vi "Date Start (000000).vi"(11 "Datetime":timestamp) -> (1 "檔名":string, 3 "Date + 00:00:00":timestamp)   [LabVIEW 2019]
panel:
  out "date string":string
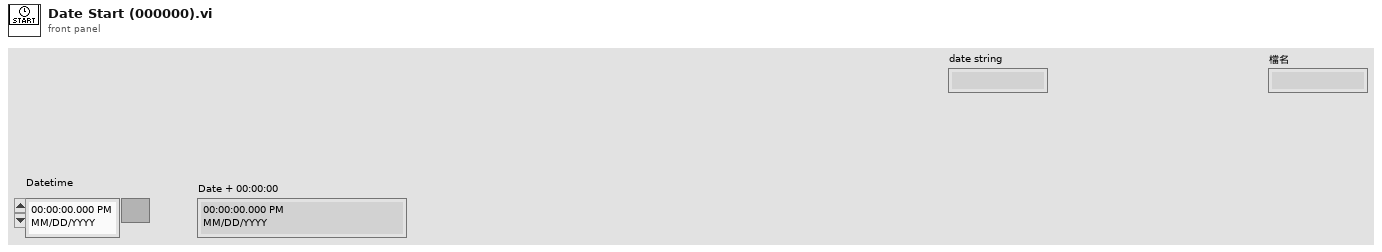
[diagram p1: front panel]
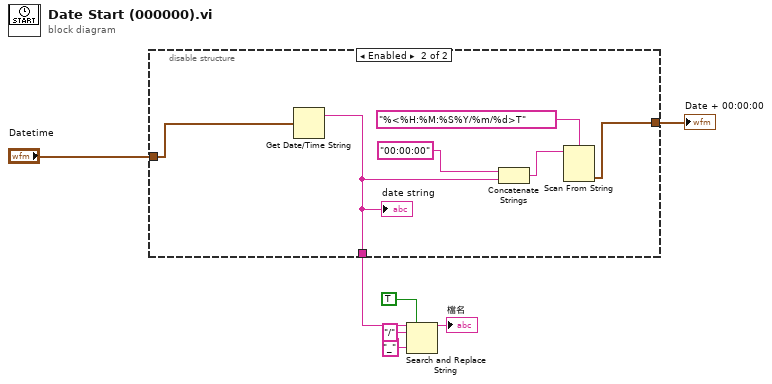
[diagram p0: block diagram]
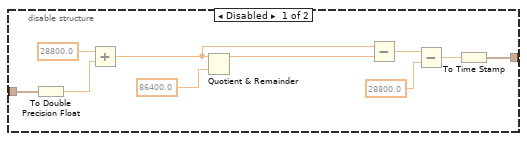
[diagram p2: hidden frame]
diagram:
  n1 = disable-structure shown="Enabled" {
    disable-tunnel: [w17 w19] -> w7
    disable-tunnel: "Datetime" -> [w8 w20]
    disable-tunnel: [_ w18] -> w5
    frame Disabled {
      n2 = To Double Precision Float(number=w8) -> (double precision float=w11:dbl)
      n3 = Add(x=28800.0, y=w11) -> (x+y=w10:dbl)
      n4 = Quotient & Remainder(x=w10, y=86400.0) -> (x-y*floor(x/y)=w9:dbl)  [unwired: 1 out]
      n5 = Subtract(x=w10, y=w9) -> (x-y=w13:dbl)
      n6 = Subtract(x=w13, y=28800.0) -> (x-y=w14:dbl)
      n7 = To Time Stamp(1:w14) -> (0:w17:timestamp)
    }
    frame Enabled {
      n8 = Get Date/Time String(seconds (now)=w20) -> (date string=w18:string)  [unwired: 2 in, 1 out]
      "date string" <- w18
      n9 = Concatenate Strings("00:00:00", w18) -> (w23:string)
      n10 = Scan From String(format string="%<%H:%M:%S%Y/%m/%d>T", input string=w23) -> (output 1=w19:timestamp)  [unwired: 3 in, 3 out]
    }
  }
  "Date + 00:00:00" <- w7
  n11 = Search and Replace String(replace all?=TRUE ("replace all? (F)"), input string=w5, search string="/", replace string="_" ("replace string (\"\")")) -> (result string=→"檔名":string)  [unwired: 4 in, 3 out]
